vi "C2LVstring.vi"(4 "CString":u8[](array[numeric])) -> (1 "LVString":string)   [LabVIEW 2019]
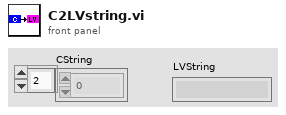
[diagram p1: front panel]
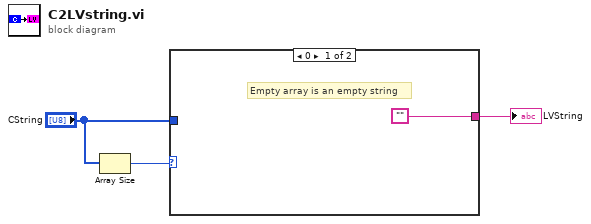
[diagram p0: block diagram]
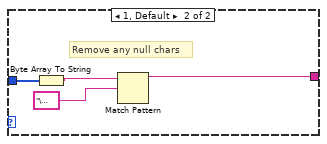
[diagram p2: hidden frame]
diagram:
  n1 = Array Size(array="CString") -> (size(s)=w3:i32)
  n2 = case shown="0" w3 {
    tunnel: ["" w5] -> w1
    tunnel: "CString" -> [_ w8]
    frame 0 {
      # "Empty array is an empty string"
    }
    frame 1, Default {
      # "Remove any null chars"
      n3 = Byte Array To String(unsigned byte array=w8) -> (string=w7:string)
      n4 = Match Pattern(string=w7, regular expression="\u0000") -> (before substring=w5:string)  [unwired: 1 in, 3 out]
    }
  }
  "LVString" <- w1
